vi "citire salvare date.vi"(8 "NN- Trained file name":path, 11 "Dataset folder":path) -> (0 "RN outputs":i32, 1 "DataSet Trainded data":path, 2 "Inputs":i32, 3 "DataSet File":path[][](array[path]), 4 "nume clase":string[](array[string]))   [LabVIEW 2024]
uses:
  <vilib>/picture/picture.llb/imagedata.ctl
  <vilib>/National Instruments/NI Super Simple Neural Networks/Types/Teaching Vector.ctl
  <vilib>/National Instruments/NI Super Simple Neural Networks/Types/1D Array.ctl
  <vilib>/National Instruments/NI Super Simple Neural Networks/Neural Network.lvclass
panel:
  out "image data":T1
  out "appended path":path
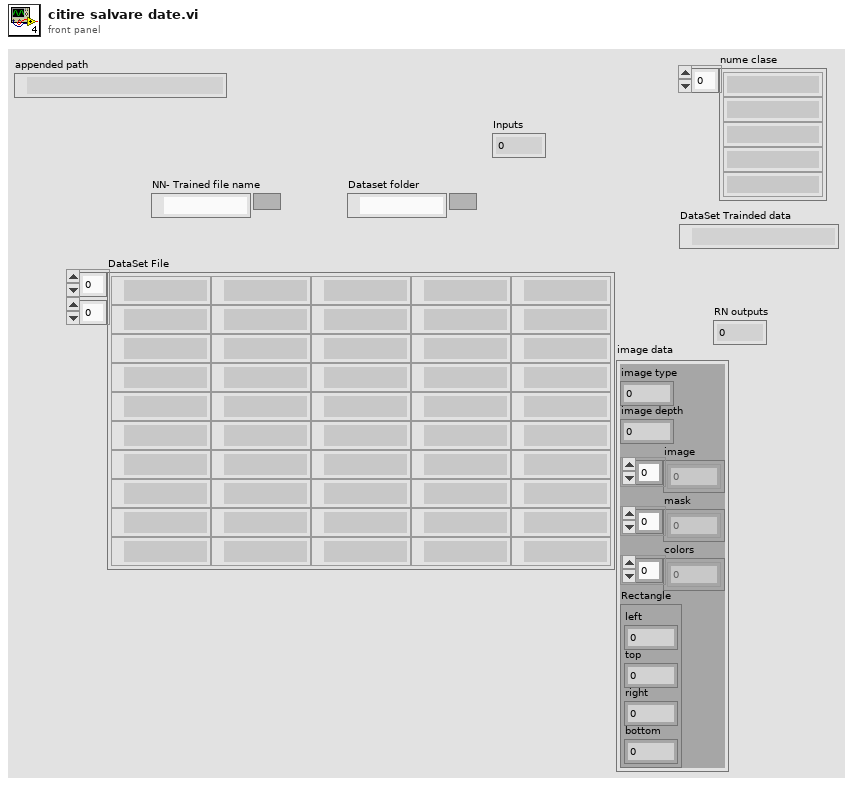
[diagram p1: front panel]
types:
  T1 = typedef "imagedata.ctl" = cluster{"image type":i32, "image depth":i32, "image":u8[], "mask":u8[], "colors":u32[], "Rectangle":cluster{"left":i16, "top":i16, "right":i16, "bottom":i16}}
  T2 = enum16{"open", "replace", "create", "open or create", "replace or create", "replace or create with confirmation"}
  T3 = typedef "Neural Network.lvclass/Teaching Vector.ctl" = cluster{"Inputs":T4, "Expected Outputs":T4}
  T4 = typedef "Neural Network.lvclass/1D Array.ctl" = cluster{"1D Array":dbl[]}
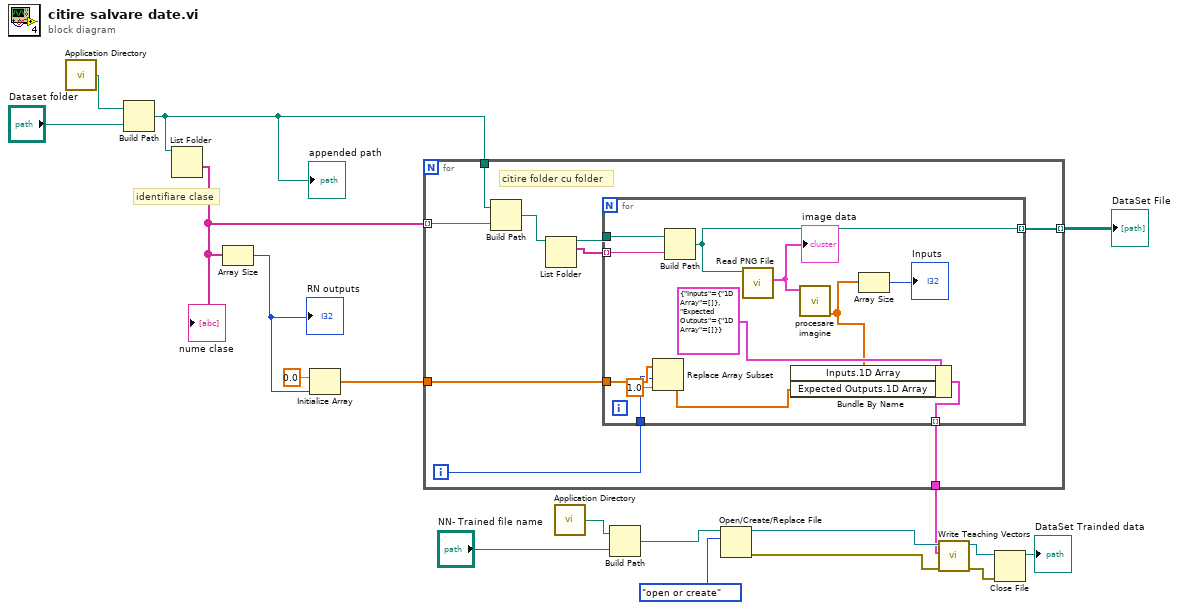
[diagram p0: block diagram]
diagram:
  # "identifiare clase"
  n1 = call <vilib>:"Application Directory.vi"() -> ("Application Directory"=w18:path)
  n2 = Build Path(base path=w18, name or relative path="Dataset folder") -> (appended path=w1:path)
  "appended path" <- w1
  n3 = List Folder(path=w1) -> (folder names=w14:string[])  [unwired: 3 in, 3 out]
  "nume clase" <- w14
  n4 = Array Size(array=w14) -> (size(s)=w16:i32)
  "RN outputs" <- w16
  n5 = Initialize Array(0.0 ("element"), w16) -> (w13:dbl[])
  n6 = for {
    tunnel: w1 -> [w27]
    tunnel: w14 -> [w26] mode=indexing
    tunnel: w13 -> [w24]
    tunnel: [w22] -> w6
    tunnel: [w21] -> w2 mode=indexing
    i -> [w23]
    # "citire folder cu folder"
    n7 = Build Path(base path=w27, name or relative path=w26) -> (appended path=w20:path)
    n8 = List Folder(path=w20) -> (path out=w25:path, filenames=w19:string[])  [unwired: 3 in, 2 out]
    n9 = for {
      tunnel: w25 -> [w39]
      tunnel: w24 -> [w37]
      tunnel: w23 -> [w36]
      tunnel: [w32] -> w22 mode=indexing
      tunnel: [w31] -> w21 mode=indexing
      tunnel: w19 -> [w28] mode=indexing
      n10 = Replace Array Subset(array=w37, new element=1.0 ("new element/subarray"), index=w36) -> (w34:dbl[])
      n11 = Build Path(base path=w39, name or relative path=w28) -> (appended path=w31:path)
      n12 = call <vilib>:"Read PNG File.vi"("path to PNG file"=w31) -> ("image data"=w38:T1)  [unwired: 8 in, 2 out]
      "image data" <- w38
      n13 = call "procesare imagine.vi"("image data"=w38) -> ("image array"=w30:sgl[])  [unwired: 9 in, 1 out]
      n14 = Bundle By Name(cluster=T3 {"Inputs"={"1D Array"=[]}, "Expected Outputs"={"1D Array"=[]}} ("Teaching Vector"), "Inputs.1D Array"=w30, "Expected Outputs.1D Array"=w34) -> (w32:T3)
      n15 = Array Size(array=w30) -> (size(s)=→"Inputs":i32)
    }
  }
  "DataSet File" <- w2
  n16 = call <vilib>:"Application Directory.vi"() -> ("Application Directory"=w12:path)
  n17 = Build Path(base path=w12, name or relative path="NN- Trained file name") -> (appended path=w10:path)
  n18 = Open/Create/Replace File(file path (use dialog)=w10, operation (0:open)=T2."open or create") -> (refnum out=w7:refnum<file>, error out=w8:errorcluster)  [unwired: 4 in, 1 out]
  n19 = call <vilib>:"Write Teaching Vectors.vi"("Error In"=w8, "Teaching Vectors"=w6, "Teaching File Ref In"=w7) -> ("Error Out"=w4:errorcluster, "Teaching File Ref Out"=w5:refnum<file>)  [unwired: 7 in]
  n20 = Close File(refnum=w5, error in=w4) -> (path=→"DataSet Trainded data":path)  [unwired: 1 out]
